vi "message scheduler trial.vi"() -> ()   [LabVIEW 2018]
uses:
  RT/Message Scheduler/Message scheduler.lvlib
  RT/Queue VIs/Queues.lvlib
  RT/Queue VIs/De-queue RT message element.vi
  RT/Message Scheduler/New infinite timed message.vi
  RT/Message Scheduler/Cancel scheduled message.vi
  RT/Message Scheduler/Quit message scheduler.vi
  Chris VIs/Message Scheduler/message scheduler.lvclass
panel:
  in  "Cancel":bool
  in  "Send":bool
  out "Iteration":i32
  out "Received string":string
  out "Schedule ID":u32
  in  "Test message":string
  in  "Quit":bool
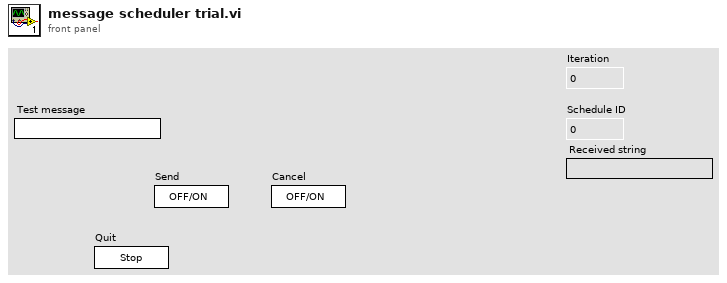
[diagram p1: front panel]
types:
  T1 = typedef "Real-Time.lvlib/Queues.lvlib/Queues cluster.ctl" = cluster{"RT Message":refnum<queue>, "RT Comms":refnum<queue>, "RT Data":refnum<queue>, "message scheduler":refnum<class "message scheduler.lvclass">}
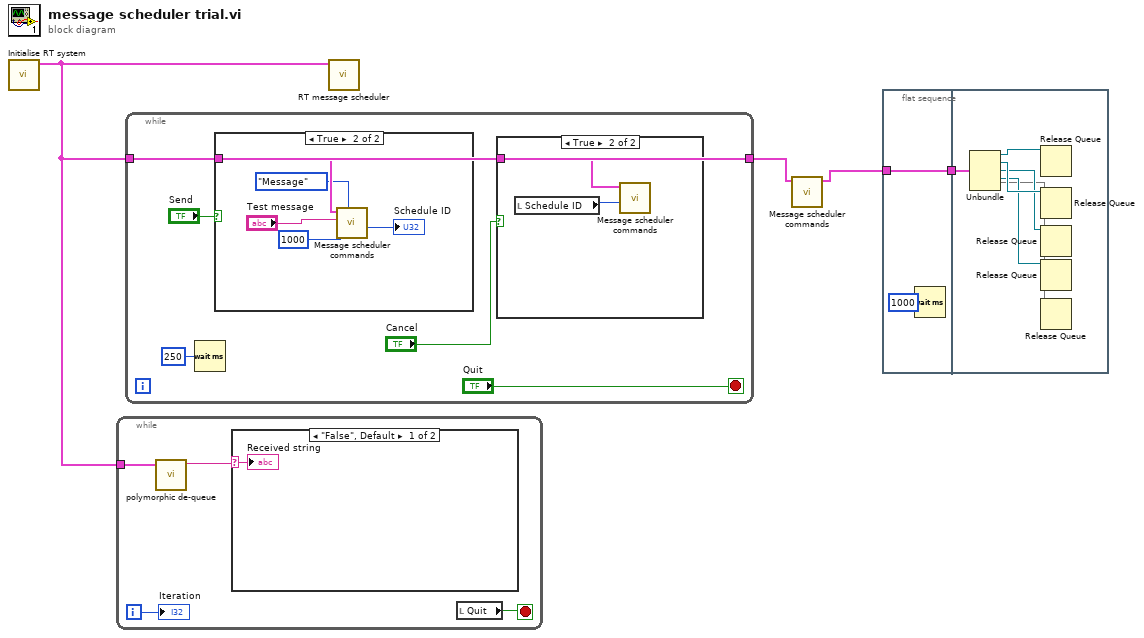
[diagram p0: block diagram]
diagram:
  n1 = call "Initialise RT system.vi"() -> ("Queues"=w4:T1)  [unwired: 11 in]
  n2 = while {
    tunnel: w4 -> [w7]
    i -> [w5]
    stop <- w8 stop-if-true
    n3 = call-poly "polymorphic de-queue.vi"("RT Queues"=w7) -> ("Message"=w6:string)  [unwired: 9 in, 1 out]
    n4 = case shown="\"False\", Default" w6 {
      selector: w6 -> [w9 _]
      frame "False", Default {
        "Received string" <- w9
      }
      frame "True" {
      }
    }
    n5 = local read "Quit"() -> (w8:bool)
    "Iteration" <- w5
  }
  n6 = while {
    tunnel: w4 -> [w11]
    tunnel: [w11] -> w3
    stop <- "Quit" stop-if-true
    n7 = Wait (ms)(milliseconds to wait=u32 250) -> ()  [unwired: 1 out]
    n8 = case shown="True" "Send" {
      tunnel: w11 -> [_ w21]
      frame False {
      }
      frame True {
        n9 = call-poly "Message scheduler commands.vi"("Target Queue"=enum16{"Message", "Comms"}."Message", "Period (ms)"=u32 1000, "Message"="Test message", "RT Queues"=w21) -> ("Schedule ID"=→"Schedule ID":u32)  [unwired: 6 in, 1 out]
      }
    }
    n10 = case shown="True" "Cancel" {
      tunnel: w11 -> [_ w16]
      frame False {
      }
      frame True {
        n11 = local read "Schedule ID"() -> (w15:u32)
        n12 = call-poly "Message scheduler commands.vi"("Schedule ID"=w15, "RT Queues"=w16) -> ()  [unwired: 9 in, 1 out]
      }
    }
  }
  n13 = call "RT message scheduler.vi"("RT Queues"=w4) -> ()  [unwired: 11 in]
  n14 = call-poly "Message scheduler commands.vi"("RT Queues"=w3) -> ("RT Queues out"=w2:T1)  [unwired: 10 in]
  n15 = flat-sequence {
    tunnel: w2 -> [w23]
    tunnel: [w23] -> w1
    tunnel: w1 -> [w24]
    frame #0 {
      n16 = Wait (ms)(milliseconds to wait=u32 1000) -> ()  [unwired: 1 out]
    }
    frame #1 {
      n17 = Unbundle(w24) -> (w29:refnum<queue>, w28:refnum<queue>, w27:refnum<queue>, w26:refnum<class "message scheduler.lvclass">, w25)
      n18 = Release Queue(queue=w29) -> ()  [unwired: 2 in, 3 out]
      n19 = Release Queue(queue=w28) -> ()  [unwired: 2 in, 3 out]
      n20 = Release Queue(queue=w27) -> ()  [unwired: 2 in, 3 out]
      n21 = Release Queue(queue=w26) -> ()  [unwired: 2 in, 3 out]
      n22 = Release Queue(queue=w25) -> ()  [unwired: 2 in, 3 out]
    }
  }
